vi "Start Bus Monitor.vi"(8 "error in (no error)":errorcluster, 10 "MediatorBusMonitor (Type)":refnum<class "IMediatorBusMonitor.lvclass">, 11 "Mediator in":refnum<class "Mediator.lvclass">) -> (0 "error out":errorcluster, 3 "Mediator out":refnum<class "Mediator.lvclass">)   [LabVIEW 2017, in "MyMediator.lvlib副本.lvlib" / "Mediator.lvclass"]
uses:
  Mediator.lvclass
  C:/Program Files (x86)/National Instruments/LabVIEW 2017/vi.lib/Composed/GPM Packages/mva-framework/Source/Framework/IMediator/IMediator/IMediator.lvclass
  <vilib>/Composed/GPM Packages/mva-framework/Source/Framework/IMediator/IMediatorBusMonitor/IMediatorBusMonitor.lvclass
  Mediator.lvclass/Mediator.ctl
  <vilib>/ActorFramework/Message Enqueuer/Message Enqueuer.lvclass/Message Enqueuer.ctl
  <vilib>/ActorFramework/Message Enqueuer/Enqueue.vi
  <vilib>/ActorFramework/Stop Msg/Stop Msg.lvclass
  C:/Program Files (x86)/National Instruments/LabVIEW 2017/vi.lib/ActorFramework/Message/Message.lvclass
  <vilib>/ActorFramework/Message Priority Queue/Priority Enqueue.vi
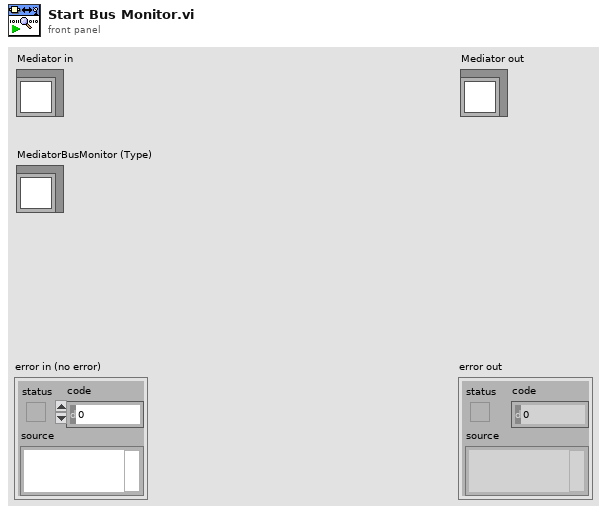
[diagram p1: front panel]
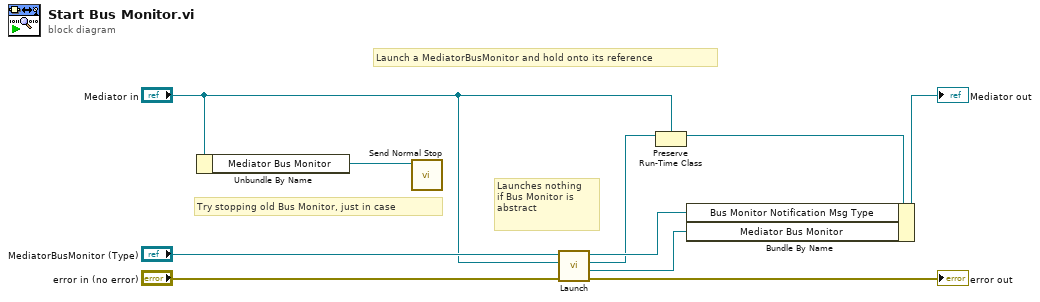
[diagram p0: block diagram]
diagram:
  # "Launches nothing\nif Bus Monitor is\nabstract"
  # "Try stopping old Bus Monitor, just in case"
  # "Launch a MediatorBusMonitor and hold onto its reference"
  n1 = Unbundle By Name("Mediator in") -> ("Mediator Bus Monitor"=w10:refnum<class "Message Enqueuer.lvclass">)
  n2 = call <vilib>:"Send Normal Stop.vi"("Message Enqueuer"=w10) -> ()  [unwired: 10 in, 1 out]
  n3 = call-dynamic "Launch.vi"("error in (no error)"="error in (no error)", "Mediator"="Mediator in", "IMediatorBusMonitor (Type)"="MediatorBusMonitor (Type)") -> ("error out"=→"error out":errorcluster, "Bus Monitor Enqueuer"=w8:refnum<class "Message Enqueuer.lvclass">, "Mediator Out"=w1:refnum<class "IMediator.lvclass">, "Notification Msg Type"=w2:refnum<class "Notification Msg.lvclass">)  [unwired: 5 in]
  n4 = Preserve Run-Time Class(object in=w1, 2:"Mediator in") -> (object out=w4:refnum<class "Mediator.lvclass">)  [unwired: 1 in, 1 out]
  n5 = Bundle By Name(cluster=w4, "Bus Monitor Notification Msg Type"=w2, "Mediator Bus Monitor"=w8) -> (→"Mediator out":refnum<class "Mediator.lvclass">)
